vi "Serialization Test.vi"() -> (0 "validation error":errorcluster, 1 "Modules Equal":bool, 2 "Pass":bool, 4 "serialization error":errorcluster, 5 "Channels Equal":bool)   [LabVIEW 2021, in "Custom Temperature Controller tests.lvlib"]
doc: "Flatten and unflatten configuration class testing the following:\n- Channels, Modules, and error classifications have nto changed after being flattened/unflattened\n- Flattening/Unflattening does not result in any errors\n- Module passes validation after serialization"
uses:
  Custom Temperature Controller tests.lvlib
  module/configuration/Custom Temperature Controller configuration.lvclass
  C:/Program Files (x86)/National Instruments/LabVIEW 2021/vi.lib/NI/DCAF/Tag Editor Core/control module/configuration/control module configuration.lvclass
  <vilib>/NI/DCAF/Tag Editor Core/control module/configuration/control module configuration.lvclass/control module configuration.ctl
  <vilib>/NI/DCAF/Tag Editor Core/control module/configuration/Read error classifications.vi
panel:
  out "Errors Equal":bool
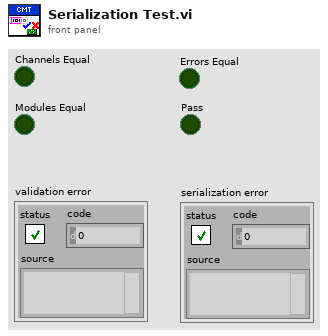
[diagram p1: front panel]
types:
  T1 = typedef "control module configuration.lvclass/error classification setting.ctl" = cluster{"code":i32, "error classification":T2}
  T2 = typedef "TBM module execution interface.lvclass/error classification.ctl" = enum16{"unknown", "none", "trivial", "recoverable", "critical"}
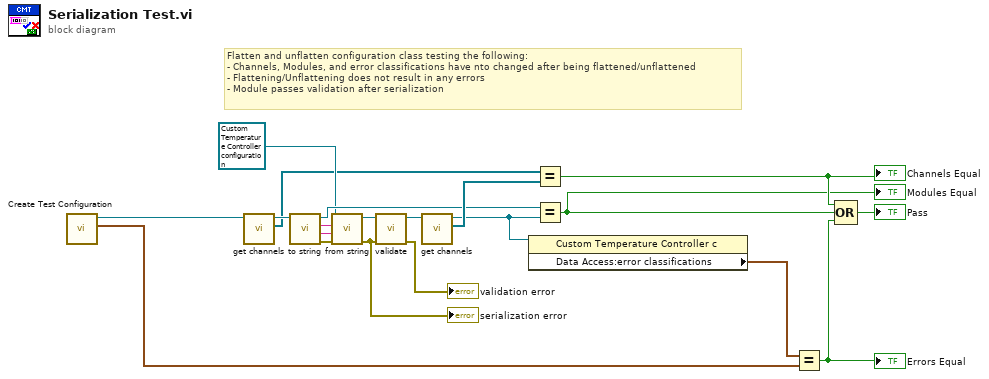
[diagram p0: block diagram]
diagram:
  # "Flatten and unflatten configuration class testing the following:\n- Channels, Modules, and error classifications have nto changed after being flattened/unflattened\n- Flattening/Unflattening does not result in any errors\n- Module passes validation after serialization"
  n1 = call "Create Test Configuration.vi"() -> ("error classifications"=w1:T1[], "Module"=w20:refnum<class "Custom Temperature Controller configuration.lvclass">)  [unwired: 6 in, 4 out]
  n2 = call-dynamic "get channels.vi"("fixed channel configuration in"=w20) -> ("channels"=w8:refnum<class "TBM channel.lvclass">[], "fixed channel configuration out"=w10:refnum<class "Custom Temperature Controller configuration.lvclass">)  [unwired: 9 in]
  n3 = call-dynamic "to string.vi"("fixed channel configuration in"=w10) -> ("error out"=w19:errorcluster, "data"=w18:string, "version"=w17:string, "fixed channel configuration out"=w11:refnum<class "Custom Temperature Controller configuration.lvclass">)  [unwired: 7 in]
  n4 = call-dynamic "from string.vi"("error in"=w19, "data"=w18, "version"=w17, "fixed channel configuration in"=refnum<class "Custom Temperature Controller configuration.lvclass"> refnum ("user control module configuration out")) -> ("error out"=w14:errorcluster, "fixed channel configuration out"=w16:refnum<class "Custom Temperature Controller configuration.lvclass">)  [unwired: 6 in]
  "serialization error" <- w14
  n5 = call-dynamic "validate.vi"("error in"=w14, "fixed channel configuration in"=w16) -> ("error out"=→"validation error":errorcluster, "fixed channel configuration out"=w13:refnum<class "Custom Temperature Controller configuration.lvclass">)  [unwired: 8 in]
  n6 = call-dynamic "get channels.vi"("fixed channel configuration in"=w13) -> ("channels"=w12:refnum<class "TBM channel.lvclass">[], "fixed channel configuration out"=w7:refnum<class "Custom Temperature Controller configuration.lvclass">)  [unwired: 9 in]
  n7 = property class="Custom Temperature Controller c"(reference=w7) -> ("Data Access:error classifications"=w6:T1[])  [unwired: 1 in, 2 out]
  n8 = Equal?(x=w8, y=w12) -> (x = y?=w5:bool)
  "Channels Equal" <- w5
  n9 = Equal?(x=w11, y=w7) -> (x = y?=w4:bool)
  "Modules Equal" <- w4
  n10 = Equal?(x=w6, y=w1) -> (x = y?=w3:bool)
  "Errors Equal" <- w3
  n11 = Compound Arithmetic op=OR(w5, w4, w3) -> (→"Pass":bool)
